vi "DMA Channel.vi"(8 "error in (no error)":errorcluster, 11 "Node Ptr":T3 format="%.0x") -> (0 "error out":errorcluster)   [LabVIEW 2016, in "FPGA Addon System Explorer.lvlib"]
uses:
  FPGA Addon System Explorer.lvlib
  <vilib>/NI Veristand/Custom Device API/Custom Device Item Ref.ctl
  Shared/Delacing Scheme.ctl
  Shared/DMA Acquisition Mode.ctl
  Shared/FG Action.ctl
  <vilib>/NI Veristand/Custom Device API/Custom Device Waveform.ctl
  <vilib>/NI Veristand/Custom Device API/Custom Device Waveform DataType.ctl
  Shared/Constants.vi
  <vilib>/NI Veristand/Custom Device API/NI VeriStand - Get Item Property.vi
  <vilib>/NI Veristand/Custom Device API/Get Item Property (U32).vi
  <vilib>/NI Veristand/Custom Device API/Get Item Property (Double).vi
  <vilib>/NI Veristand/Custom Device API/NI VeriStand - Set Item Property.vi
  <vilib>/NI Veristand/Custom Device API/Set Item Property (U32).vi
  <vilib>/NI Veristand/Custom Device API/Set Item Property (Double).vi
  <vilib>/NI Veristand/Custom Device Tools/Custom Device Utility Library/NI VeriStand - Search for All Items by GUID.vi
  <vilib>/NI VeriStand/Custom Device API/Custom Device API.lvlib
  <vilib>/NI VeriStand/Custom Device Tools/Custom Device Utility Library/Custom Device Utility Library.lvlib
  FPGA-Resource-Manager-APIs/Source/Shared/FPGA RM Shared API.lvlib
  Shared/FPGA Addon Shared.lvlib
panel:
  in  "DMA Host Buffer":u32(ring)=5 items=["1 Second"=1, "2 Seconds"=2, "5 Seconds"=5, "10 Seconds"=10]
  out "Original Name":string
  in  "Number of Samples":u32
  in  "Mode":T1
  in  "dt":dbl format="%#_p"
  in  "Reset":bool
  in  "Apply":bool
  in  "Update Rate":u32(ring)=1 items=["1 Hz"=1, "2 Hz"=2, "5 Hz"=5, "10 Hz"=10]
  in  "Delacing Scheme":T2
  in  "Number of Channels":u8
  in  "Header 2":cluster{"Section Name":string}={"Section Name"="Custom Device Item Settings"}
  in  "SHDocVw.IWebBrowser":refnum<k7>(container)
  in  "Header":cluster{"Section Name":string}={"Section Name"="Custom Device Item Settings"}
  in  "Description":string
  in  "Name":string
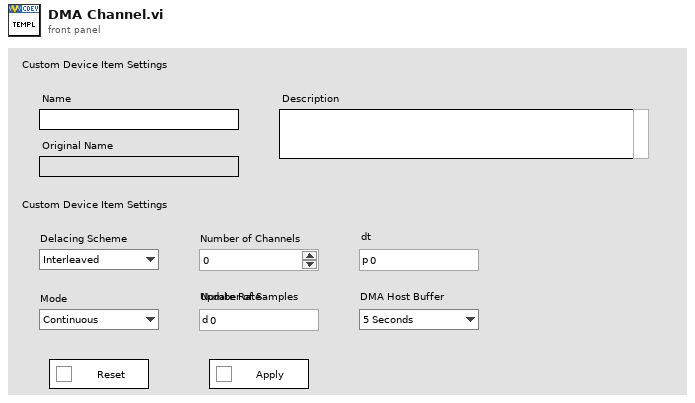
[diagram p1: front panel]
types:
  T1 = typedef "FPGA Addon Shared.lvlib/DMA Acquisition Mode.ctl" = enum8{"Continuous", "Triggered Finite"}
  T2 = typedef "FPGA Addon Shared.lvlib/Delacing Scheme.ctl" = enum8{"Interleaved"}
  T3 = typedef "Custom Device API.lvlib/Custom Device Item Ref.ctl" = u64
  T4 = typedef "Custom Device API.lvlib/Custom Device Item Info.ctl" = cluster{"Name":string, "Is Channel":bool, "GUID":string, "Is Waveform":bool}
  T5 = typedef "FPGA RM Shared API.lvlib/FG Action.ctl" = enum8{"GET", "SET"}
  T6 = typedef "FPGA Addon Shared.lvlib/DMA Settings.ctl" = cluster{"Number of Channels":u8, "Delacing Scheme":T2, "Update Rate":u32, "dt":dbl, "Mode":T1, "Number of Samples":u32, "DMA Host Buffer":u32}
  T7 = typedef "Custom Device API.lvlib/Custom Device Waveform.ctl" = cluster{"Data Type":T8, "Units":string}
  T8 = typedef "Custom Device API.lvlib/Custom Device Waveform DataType.ctl" = enum16{"Double", "Complex Double"}
  T9 = typedef "Custom Device API.lvlib/Custom Device Commands.ctl" = enum16{"Default", "Item renamed", "Shutdown", "Dynamic button pressed"}
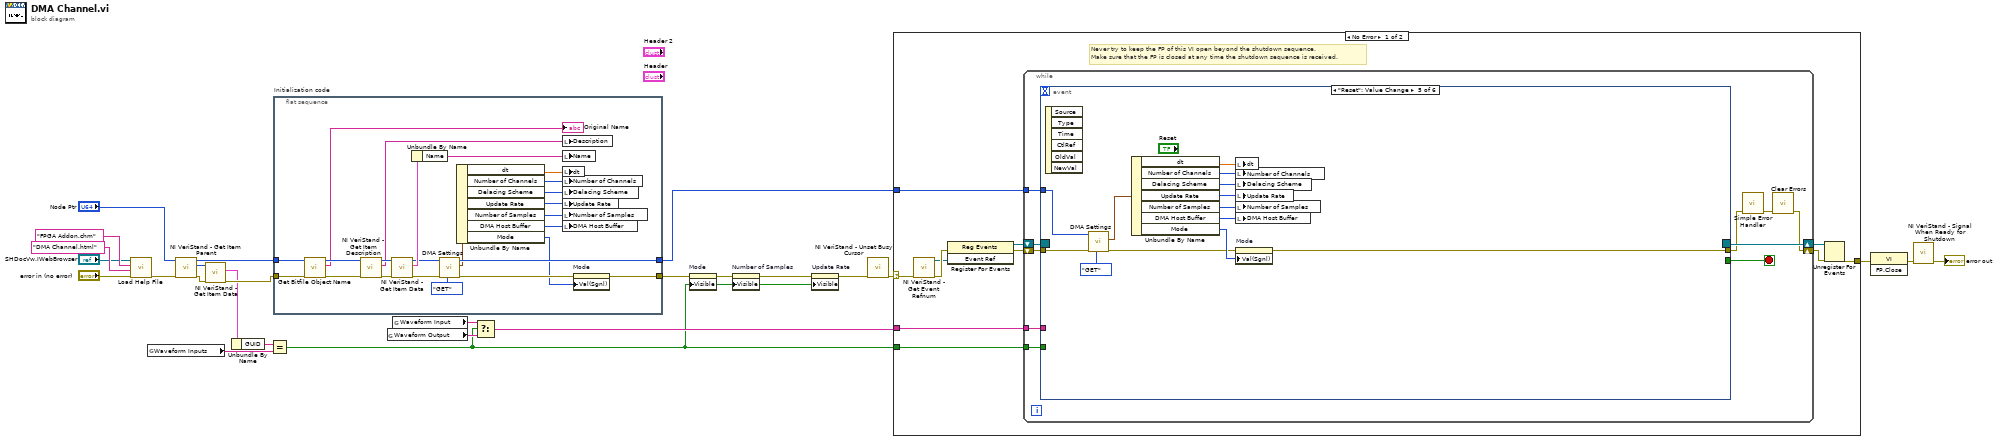
[diagram p0: block diagram]
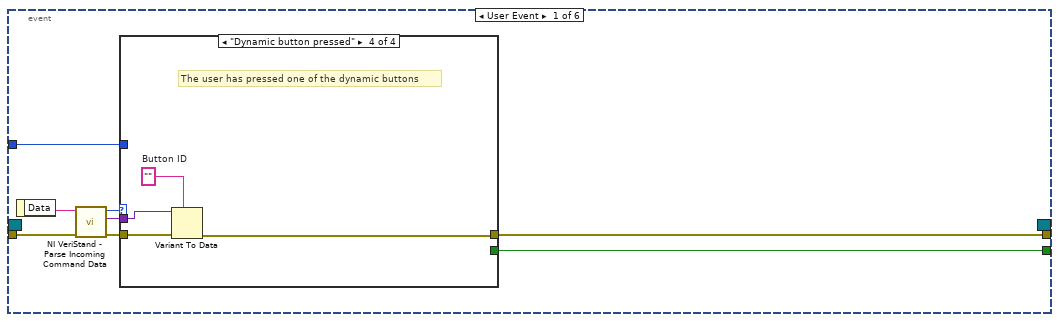
[diagram p2: hidden frame]
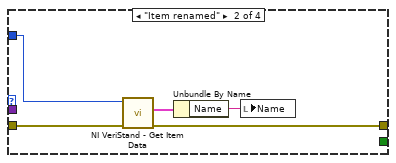
[diagram p4: hidden frame]
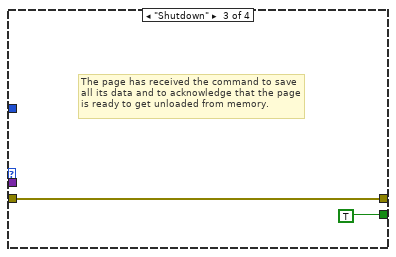
[diagram p5: hidden frame]
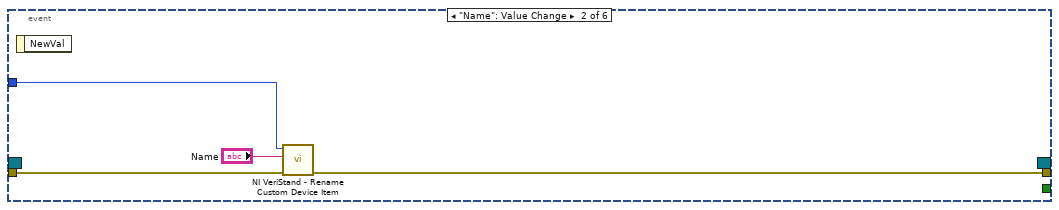
[diagram p6: hidden frame]
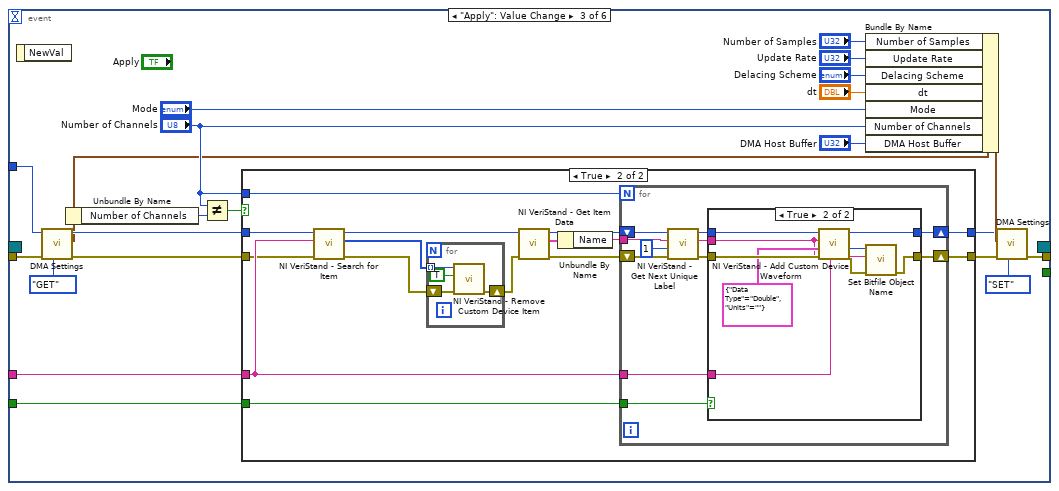
[diagram p7: hidden frame]
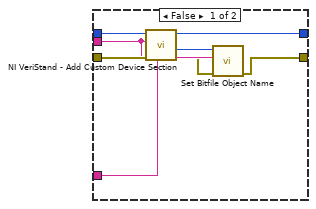
[diagram p9: hidden frame]
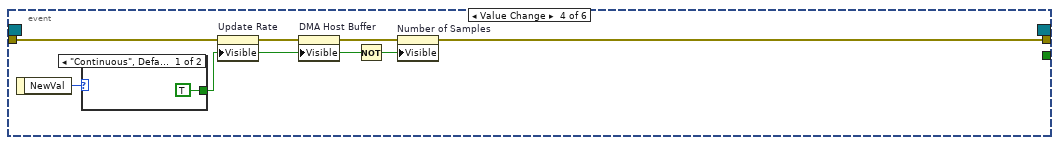
[diagram p10: hidden frame]
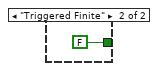
[diagram p11: hidden frame]
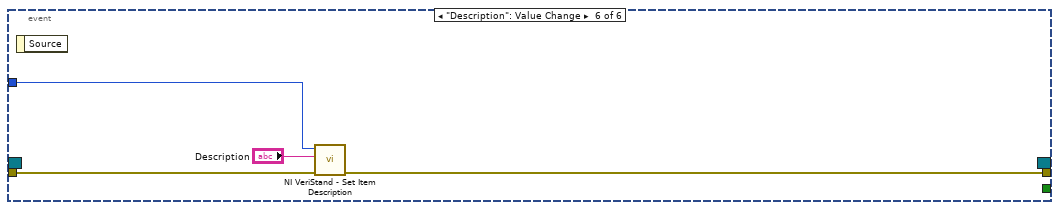
[diagram p12: hidden frame]
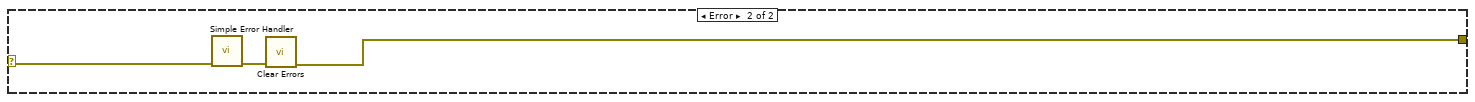
[diagram p13: hidden frame]
diagram:
  n1 = call "Load Help File.vi"("error in (no error)"="error in (no error)", "HTML File"="DMA Channel.html", "Main CHM File"="FPGA Addon.chm", "SHDocVw.IWebBrowser2"="SHDocVw.IWebBrowser") -> ("error out"=w17:errorcluster)  [unwired: 7 in]
  n2 = global read "Constants.vi" "Waveform Inputs"() -> (w9:string)
  n3 = call <vilib>:"NI VeriStand - Get Item Parent.vi"("error in (no error)"=w17, "Item Ref in"="Node Ptr") -> ("error out"=w13:errorcluster, "Parent Ref"=w14:T3, "Item Ref out"=w15:T3)  [unwired: 6 in, 1 out]
  n4 = call <vilib>:"NI VeriStand - Get Item Data.vi"("error in (no error)"=w13, "Item Ref in"=w14) -> ("error out"=w12:errorcluster, "Item Info"=w11:T4)  [unwired: 8 out]
  n5 = Unbundle By Name(w11) -> ("GUID"=w10:string)
  n6 = Equal?(x=w10, y=w9) -> (x = y?=w1:bool)
  n7 = flat-sequence "Initialization code" {
    tunnel: w12 -> [w31]
    tunnel: w15 -> [w32]
    tunnel: [w34] -> w3
    tunnel: [w43] -> w22
    frame #0 {
      n8 = call "Get Bitfile Object Name.vi"("error in (no error)"=w31, "Item Ref in"=w32) -> ("error out"=w30:errorcluster, "Value"=→"Original Name":string, "Item Ref out"=w29:T3)  [unwired: 7 in]
      n9 = call <vilib>:"NI VeriStand - Get Item Description.vi"("error in (no error)"=w30, "Item Ref in"=w29) -> ("error out"=w48:errorcluster, "Description"=w49:string, "Item Ref out"=w50:T3)  [unwired: 7 out]
      n10 = call <vilib>:"NI VeriStand - Get Item Data.vi"("error in (no error)"=w48, "Item Ref in"=w50) -> ("error out"=w45:errorcluster, "Item Info"=w47:T4, "Item Ref out"=w44:T3)  [unwired: 7 out]
      n11 = Unbundle By Name(w47) -> ("Name"=w46:string)
      n12 = call "DMA Settings.vi"("Action"=FG_Action."GET", "error in (no error)"=w45, "Item Ref"=w44) -> ("error out"=w37:errorcluster, "DMA Settings"=w41:T6, "Item Ref out"=w43:T3)  [unwired: 6 in]
      n13 = Unbundle By Name(w41) -> ("dt"=w38:dbl, "Number of Channels"=w39:u8, "Delacing Scheme"=w40:T2, "Update Rate"=w36:u32, "Number of Samples"=w35:u32, "DMA Host Buffer"=w27:u32, "Mode"=w33:T1)
      n14 = local write "Description"(w49) -> ()
      n15 = local write "Name"(w46) -> ()
      n16 = local write "dt"(w38) -> ()
      n17 = local write "Number of Channels"(w39) -> ()
      n18 = local write "Delacing Scheme"(w40) -> ()
      n19 = local write "Update Rate"(w36) -> ()
      n20 = local write "Number of Samples"(w35) -> ()
      n21 = local write "DMA Host Buffer"(w27) -> ()
      n22 = property on="Mode" class="Enum (strict)"(error in=w37, "Val(Sgnl)"=w33) -> (error out=w34:errorcluster)  [unwired: 1 in, 1 out]
    }
  }
  n23 = global read "Constants.vi" "Waveform Output"() -> (w7:string)
  n24 = global read "Constants.vi" "Waveform Input"() -> (w8:string)
  n25 = Select(t=w8, s=w1, f=w7) -> (s? t:f=w6:string)
  n26 = property on="Mode" class="Enum (strict)"(error in=w3, "Visible"=w1) -> (error out=w5:errorcluster)  [unwired: 1 in, 1 out]
  n27 = property on="Number of Samples" class="DigNum (strict)"(error in=w5, "Visible"=w1) -> (error out=w4:errorcluster)  [unwired: 1 in, 1 out]
  n28 = property on="Update Rate" class="Ring (strict)"(error in=w4, "Visible"=w1) -> (error out=w2:errorcluster)  [unwired: 1 in, 1 out]
  n29 = call <vilib>:"NI VeriStand - Unset Busy Cursor.vi"("error in (no error)"=w2) -> ("error out"=w23:errorcluster)  [unwired: 10 out]
  n30 = case shown="No Error" w23 {
    selector: w23 -> [w53 w194]
    tunnel: [w58 w192] -> w26
    tunnel: w22 -> [w54 _]
    tunnel: w6 -> [w52 _]
    tunnel: w1 -> [w51 _]
    frame No Error {
      # "Never try to keep the FP of this VI open beyond the shutdown sequence.\nMake sure that the FP is closed at any time the shutdown sequence is received."
      n31 = call <vilib>:"NI VeriStand - Get Event Refnum.vi"("error in (no error)"=w53) -> ("error out"=w61:errorcluster, "Event Ref"=w57:refnum<user-event>)  [unwired: 9 out]
      n32 = register-events(error in=w61, w57) -> (reference out=w55:refnum<event-registration>, error out=w56:errorcluster)  [unwired: 1 in]
      n33 = while {
        tunnel: w54 -> [w67]
        shift-right: [w64] -> w59
        shift-left: w56 -> [w70]
        shift-right: [w71] -> w60
        shift-left: w55 -> [w69]
        tunnel: w52 -> [w63]
        tunnel: w51 -> [w62]
        stop <- w68 stop-if-true
        n34 = event shown="[4] \"Reset\": Value Change" {
          selector: w69 -> [_ _ _ _ _ _]
          dyn-events: [_ _ _ _ _ _] -> w71
          timeout: _ -> [_ _ _ _ _ _]
          tunnel: w70 -> [w79 w95 w107 w170 w184 w190]
          tunnel: [w75 _ _ _ _ _] -> w68
          tunnel: [w74 w94 w117 w169 w176 w189] -> w66
          tunnel: w67 -> [w73 w93 w105 _ w183 w191]
          tunnel: w63 -> [_ _ w112 _ _ _]
          tunnel: w62 -> [_ _ w110 _ _ _]
          event User Event {
            n35 = event-data() -> ("Data"=w78:string)  [unwired: 1 out]
            n36 = call <vilib>:"NI VeriStand - Parse Incoming Command Data.vi"("error in (no error)"=w79, "Incoming data"=w78) -> ("error out"=w77:errorcluster, "Outgoing data"=w72:variant, "Action"=w76:T9)  [unwired: 7 out]
            n37 = case shown="\"Dynamic button pressed\"" w76 {
              tunnel: w77 -> [w80 w85 w86 w91]
              tunnel: [_ _ TRUE _] -> w75
              tunnel: [w80 w82 w86 w88] -> w74
              tunnel: w73 -> [_ w84 _ _]
              tunnel: w72 -> [_ _ _ w90]
              frame "Default", Default {
              }
              frame "Item renamed" {
                n38 = call <vilib>:"NI VeriStand - Get Item Data.vi"("error in (no error)"=w85, "Item Ref in"=w84) -> ("error out"=w82:errorcluster, "Item Info"=w83:T4)  [unwired: 8 out]
                n39 = Unbundle By Name(w83) -> ("Name"=w81:string)
                n40 = local write "Name"(w81) -> ()
              }
              frame "Shutdown" {
                # "The page has received the command to save all its data and to acknowledge that the page is ready to get unloaded from memory."
              }
              frame "Dynamic button pressed" {
                w89 = ""  # Button ID
                # "The user has pressed one of the dynamic buttons"
                n41 = Variant To Data(error in=w91, type=w89, Variant=w90) -> (error out=w88:errorcluster)  [unwired: 1 out]
              }
            }
          }
          event "Name": Value Change {
            n42 = event-data() -> ()  [unwired: 2 out]
            n43 = call <vilib>:"NI VeriStand - Rename Custom Device Item.vi"("error in (no error)"=w95, "New Name"="Name", "Item Ref in"=w93) -> ("error out"=w94:errorcluster)  [unwired: 1 in, 7 out]
          }
          event "Apply": Value Change {
            n44 = event-data() -> ()  [unwired: 2 out]
            n45 = call "DMA Settings.vi"("Action"=FG_Action."GET", "error in (no error)"=w107, "Item Ref"=w105) -> ("error out"=w106:errorcluster, "DMA Settings"=w99:T6, "Item Ref out"=w104:T3)  [unwired: 6 in]
            n46 = Unbundle By Name(w99) -> ("Number of Channels"=w103:u8)
            n47 = Not Equal?(x="Number of Channels", y=w103) -> (x != y?=w100:bool)
            n48 = case shown="True" w100 {
              tunnel: w112 -> [_ w126]
              tunnel: w110 -> [_ w125]
              tunnel: [w118 w124] -> w109
              tunnel: w106 -> [w118 w123]
              tunnel: w104 -> [w119 w122]
              tunnel: "Number of Channels" -> [_ w121]
              tunnel: [w119 w120] -> w101
              frame False {
              }
              frame True {
                n49 = call-poly <vilib>:"NI VeriStand - Search for Item.vi"("Item GUID"=w126, "Section Ref in"=w122) -> ("Item Refs"=w128:T3[], "Section Ref out"=w129:T3)  [unwired: 6 in, 2 out]
                n50 = for {
                  tunnel: w128 -> [w137] mode=indexing
                  shift-right: [w135] -> w127
                  shift-left: w123 -> [w136]
                  n51 = call <vilib>:"NI VeriStand - Remove Custom Device Item.vi"("error in (no error)"=w136, "Force Delete (F)"=TRUE, "Item Ref in"=w137) -> ("error out"=w135:errorcluster)  [unwired: 7 in, 1 out]
                }
                n52 = call <vilib>:"NI VeriStand - Get Item Data.vi"("error in (no error)"=w127, "Item Ref in"=w129) -> ("error out"=w133:errorcluster, "Item Info"=w131:T4, "Item Ref out"=w132:T3)  [unwired: 7 out]
                n53 = Unbundle By Name(w131) -> ("Name"=w130:string)
                n54 = for {
                  N: w121 -> [_]
                  tunnel: w130 -> [w142]
                  shift-right: [w148] -> w124
                  shift-left: w133 -> [w144]
                  shift-right: [w140] -> w120
                  shift-left: w132 -> [w143]
                  tunnel: w126 -> [w139]
                  tunnel: w125 -> [w138]
                  n55 = call <vilib>:"NI VeriStand - Get Next Unique Label.vi"("error in (no error)"=w144, "Start Value (1)"=1, "Label"=w142, "Parent Ref in"=w143) -> ("error out"=w147:errorcluster, "Label out"=w145:string, "Parent Ref dup"=w146:T3)  [unwired: 4 in, 1 out]
                  n56 = case shown="True" w138 {
                    tunnel: [w149 w157] -> w148
                    tunnel: w147 -> [w155 w165]
                    tunnel: w146 -> [w156 w164]
                    tunnel: w145 -> [w151 w159]
                    tunnel: [w153 w162] -> w140
                    tunnel: w139 -> [w154 w161]
                    frame False {
                      n57 = call <vilib>:"NI VeriStand - Add Custom Device Section.vi"("GUID (Default Section)"=w154, "error in (no error)"=w155, "Section Name"=w151, "Parent Ref in"=w156) -> ("error out"=w150:errorcluster, "Section Ptr"=w152:T3, "Parent Ref out"=w153:T3)  [unwired: 4 in, 1 out]
                      n58 = call "Set Bitfile Object Name.vi"("error in (no error)"=w150, "Name"=w151, "Channel Ref"=w152) -> ("error out"=w149:errorcluster)  [unwired: 8 in]
                    }
                    frame True {
                      n59 = call <vilib>:"NI VeriStand - Add Custom Device Waveform.vi"("GUID (Default Waveform)"=w161, "error in (no error)"=w165, "Waveform"=T7 {"Data Type"=enum."Double", "Units"=""}, "Waveform Name"=w159, "Parent Ref in"=w164) -> ("error out"=w158:errorcluster, "Waveform Ref"=w160:T3, "Parent Ref out"=w162:T3)  [unwired: 3 in, 1 out]
                      n60 = call "Set Bitfile Object Name.vi"("error in (no error)"=w158, "Name"=w159, "Channel Ref"=w160) -> ("error out"=w157:errorcluster)  [unwired: 8 in]
                    }
                  }
                }
              }
            }
            n61 = Bundle By Name(cluster=w99, "Number of Samples"="Number of Samples", "Update Rate"="Update Rate", "Delacing Scheme"="Delacing Scheme", "dt"="dt", "Mode"="Mode", "Number of Channels"="Number of Channels", "DMA Host Buffer"="DMA Host Buffer") -> (w113:T6)
            n62 = call "DMA Settings.vi"("Action"=FG_Action."SET", "error in (no error)"=w109, "DMA Settings"=w113, "Item Ref"=w101) -> ("error out"=w117:errorcluster)  [unwired: 5 in, 2 out]
          }
          event Value Change {
            n63 = event-data() -> ("NewVal"=w171:T1)  [unwired: 1 out]
            n64 = case shown="\"Continuous\", Default" w171 {
              tunnel: [TRUE FALSE] -> w166
              frame "Continuous", Default {
              }
              frame "Triggered Finite" {
              }
            }
            n65 = property on="Update Rate" class="Ring (strict)"(error in=w170, "Visible"=w166) -> (error out=w168:errorcluster)  [unwired: 1 in, 1 out]
            n66 = property on="DMA Host Buffer" class="Ring (strict)"(error in=w168, "Visible"=w166) -> (error out=w167:errorcluster)  [unwired: 1 in, 1 out]
            n67 = Not(x=w166) -> (.not. x?=w172:bool)
            n68 = property on="Number of Samples" class="DigNum (strict)"(error in=w167, "Visible"=w172) -> (error out=w169:errorcluster)  [unwired: 1 in, 1 out]
          }
          event "Reset": Value Change {
            n69 = event-data() -> ()  [unwired: 7 out]
            n70 = call "DMA Settings.vi"("Action"=FG_Action."GET", "error in (no error)"=w184, "Item Ref"=w183) -> ("error out"=w177:errorcluster, "DMA Settings"=w182:T6)  [unwired: 6 in, 1 out]
            n71 = Unbundle By Name(w182) -> ("dt"=w180:dbl, "Number of Channels"=w181:u8, "Delacing Scheme"=w186:T2, "Update Rate"=w187:u32, "Number of Samples"=w178:u32, "DMA Host Buffer"=w175:u32, "Mode"=w179:T1)
            n72 = local write "dt"(w180) -> ()
            n73 = local write "Number of Channels"(w181) -> ()
            n74 = local write "Delacing Scheme"(w186) -> ()
            n75 = local write "Update Rate"(w187) -> ()
            n76 = local write "Number of Samples"(w178) -> ()
            n77 = local write "DMA Host Buffer"(w175) -> ()
            n78 = property on="Mode" class="Enum (strict)"(error in=w177, "Val(Sgnl)"=w179) -> (error out=w176:errorcluster)  [unwired: 1 in, 1 out]
          }
          event "Description": Value Change {
            n79 = event-data() -> ()  [unwired: 2 out]
            n80 = call <vilib>:"NI VeriStand - Set Item Description.vi"("error in (no error)"=w190, "Description"="Description", "Item Ref in"=w191) -> ("error out"=w189:errorcluster)  [unwired: 8 out]
          }
        }
        n81 = call <vilib>:"Simple Error Handler.vi"("error in (no error)"=w66) -> ("error out"=w65:errorcluster)  [unwired: 1 in, 7 out]
        n82 = call <vilib>:"Clear Errors.vi"("error in (no error)"=w65) -> ("error out"=w64:errorcluster)  [unwired: 1 in, 5 out]
      }
      n83 = Unregister For Events(event registration refnum=w60, error in=w59) -> (error out=w58:errorcluster)
    }
    frame Error {
      n84 = call <vilib>:"Simple Error Handler.vi"("error in (no error)"=w194) -> ("error out"=w193:errorcluster)  [unwired: 1 in, 7 out]
      n85 = call <vilib>:"Clear Errors.vi"("error in (no error)"=w193) -> ("error out"=w192:errorcluster)  [unwired: 1 in, 5 out]
    }
  }
  n86 = invoke class="VI" method="FP.Close"(error in=w26) -> (error out=w25:errorcluster)  [unwired: 2 in, 2 out]
  n87 = call <vilib>:"NI VeriStand - Signal When Ready for Shutdown.vi"("error in (no error)"=w25) -> ("error out"=→"error out":errorcluster)  [unwired: 10 out]
